vi "StreamProcess.Main.vi"(8 "error in (no error)":errorcluster, 9 "Refs":T1, 10 "FilterDVR.Ref":refnum<data-value>, 11 "Settings":T3) -> (0 "error out":errorcluster)   [LabVIEW 2025, in "xnet_can_bus_monitor_api_server_do.lvlib"]
uses:
  xnet_can_bus_monitor_api_server_do.lvlib
  Types/XNET.InitialSettings.ctl
  xnet_can_bus_monitor_api_server/RPC Messages/ni_xnet_can_bm_api_ConnectSettings.ctl
  xnet_can_bus_monitor_api_server/RPC Messages/ni_xnet_can_bm_api_CanMode.ctl
  xnet_can_bus_monitor_api_server/RPC Messages/ni_xnet_can_bm_api_Termination.ctl
  xnet_can_bus_monitor_api_server/RPC Messages/ni_xnet_can_bm_api_FdIsoMode.ctl
  xnet_can_bus_monitor_api_server/RPC Messages/ni_xnet_can_bm_api_FilterInfo.ctl
  xnet_can_bus_monitor_api_server/RPC Messages/ni_xnet_can_bm_api_DirectionFilter.ctl
  xnet_can_bus_monitor_api_server/RPC Messages/ni_xnet_can_bm_api_FrameFilter.ctl
  Types/StreamProcess.InputRefs.ctl
  <vilib>/gRPC/LabVIEW gRPC Library/Shared/grpcId.ctl
  Types/StreamProcess.State.ctl
  xnet_can_bus_monitor_api_server/RPC Messages/ni_xnet_can_bm_api_StreamBusReply.ctl
  xnet_can_bus_monitor_api_server/RPC Messages/ni_xnet_can_bm_api_CanCommState.ctl
  xnet_can_bus_monitor_api_server/RPC Messages/ni_xnet_can_bm_api_CommState.ctl
  xnet_can_bus_monitor_api_server/RPC Messages/ni_xnet_can_bm_api_LastCommError.ctl
  xnet_can_bus_monitor_api_server/RPC Messages/ni_xnet_can_bm_api_Frame.ctl
  xnet_can_bus_monitor_api_server/RPC Messages/ni_xnet_can_bm_api_ErrorInfo.ctl
  <vilib>/xnet/xnet.llb/XNET Create Session (Frame Input Stream).vi
  <vilib>/Utility/SystemLogging/Write to System Log.vi
  <vilib>/xnet/xnet.llb/XNET Read (Frame CAN).vi
  <vilib>/xnet/xnet.llb/XNET Read (State CAN Comm).vi
  <resource>/objmgr/xnet.rc
  xnet_can_bus_monitor_api_server/xnet_can_bus_monitor_api_server.lvlib
  xnet_can_bus_monitor_api_server/RPC Service/NI_XNET_CAN_Bus_Monitor_API/NI_XNET_CAN_Bus_Monitor_API.lvclass
  <vilib>/gRPC/LabVIEW gRPC Library/grpc-lvsupport-release.lvlib
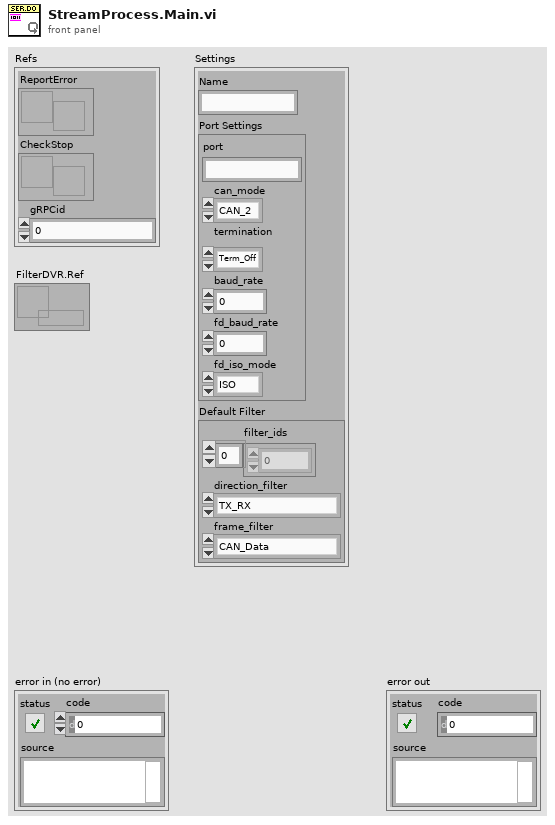
[diagram p1: front panel]
types:
  T1 = typedef "xnet_can_bus_monitor_api_server_do.lvlib/StreamProcess.InputRefs.ctl" = cluster{"ReportError":refnum<notifier>, "CheckStop":refnum<notifier>, "gRPCid":T2}
  T2 = typedef "grpc-lvsupport-release.lvlib/grpcId.ctl" = u64
  T3 = typedef "xnet_can_bus_monitor_api_server_do.lvlib/XNET.InitialSettings.ctl" = cluster{"Name":string, "Port Settings":T4, "Default Filter":T8}
  T4 = typedef "xnet_can_bus_monitor_api_server.lvlib/ni_xnet_can_bm_api_ConnectSettings.ctl" = cluster{"port":string, "can_mode":T5, "termination":T6, "baud_rate":u64, "fd_baud_rate":u64, "fd_iso_mode":T7}
  T5 = typedef "xnet_can_bus_monitor_api_server.lvlib/ni_xnet_can_bm_api_CanMode.ctl" = enum32{"CAN_2", "CAN_FD", "CAN_FD_BRS"}
  T6 = typedef "xnet_can_bus_monitor_api_server.lvlib/ni_xnet_can_bm_api_Termination.ctl" = enum32{"Term_Off", "Term_On"}
  T7 = typedef "xnet_can_bus_monitor_api_server.lvlib/ni_xnet_can_bm_api_FdIsoMode.ctl" = enum32{"ISO", "Non_ISO", "ISO_Legacy"}
  T8 = typedef "xnet_can_bus_monitor_api_server.lvlib/ni_xnet_can_bm_api_FilterInfo.ctl" = cluster{"filter_ids":u32[], "direction_filter":T9, "frame_filter":T10}
  T9 = typedef "xnet_can_bus_monitor_api_server.lvlib/ni_xnet_can_bm_api_DirectionFilter.ctl" = enum32{"TX_RX", "RX", "TX"}
  T10 = typedef "xnet_can_bus_monitor_api_server.lvlib/ni_xnet_can_bm_api_FrameFilter.ctl" = enum32{"CAN_Data", "CAN_Remote", "CAN_Bus_Error", "CAN_2_Data", "CAN_FD_Data", "CAN_FD_BRS_Data", "J1939_Data", "Delay", "Log_Trigger", "Start_Trigger", "All"}
  T11 = typedef "xnet_can_bus_monitor_api_server_do.lvlib/StreamProcess.State.ctl" = enum8{"Open XNET Session", "Publish", "Cleanup"}
  T12 = typedef "xnet_can_bus_monitor_api_server.lvlib/ni_xnet_can_bm_api_StreamBusReply.ctl" = cluster{"can_comm_state":T13, "frame":T16[], "error":T17}
  T13 = typedef "xnet_can_bus_monitor_api_server.lvlib/ni_xnet_can_bm_api_CanCommState.ctl" = cluster{"fault_code":i32, "fault":bool, "comm_state":T14, "last_comm_error":T15, "receive_error_counter":u32, "transmit_error_counter":u32, "transceiver_error":bool, "sleep":bool}
  T14 = typedef "xnet_can_bus_monitor_api_server.lvlib/ni_xnet_can_bm_api_CommState.ctl" = enum32{"Error_Active", "Error_Passive", "Bus_Off", "Init"}
  T15 = typedef "xnet_can_bus_monitor_api_server.lvlib/ni_xnet_can_bm_api_LastCommError.ctl" = enum32{"None", "Stuff", "Form", "ACK", "Bit1", "Bit0", "CRC"}
  T16 = typedef "xnet_can_bus_monitor_api_server.lvlib/ni_xnet_can_bm_api_Frame.ctl" = cluster{"timestamp":dbl, "payload":u8[], "identifier":u32, "frame_type":u32, "extended":bool, "echo":bool}
  T17 = typedef "xnet_can_bus_monitor_api_server.lvlib/ni_xnet_can_bm_api_ErrorInfo.ctl" = errorcluster
  T18 = typedef "XNET Frame CAN.ctl" = cluster{"timestamp":timestamp, "payload":u8[], "identifier":u32, "type":T19, "extended?":bool, "echo?":bool}
  T19 = typedef "XNET Frame Type CAN.ctl" = u8
  T20 = typedef "XNET CAN Comm.ctl" = cluster{"fault code":i32, "fault?":bool, "communication state":T21, "last error":T22, "receive error counter":u8, "transmit error counter":u8, "transceiver error?":bool, "sleep?":bool}
  T21 = typedef "XNET CAN Comm State.ctl" = u8
  T22 = typedef "XNET CAN Last Err.ctl" = u8
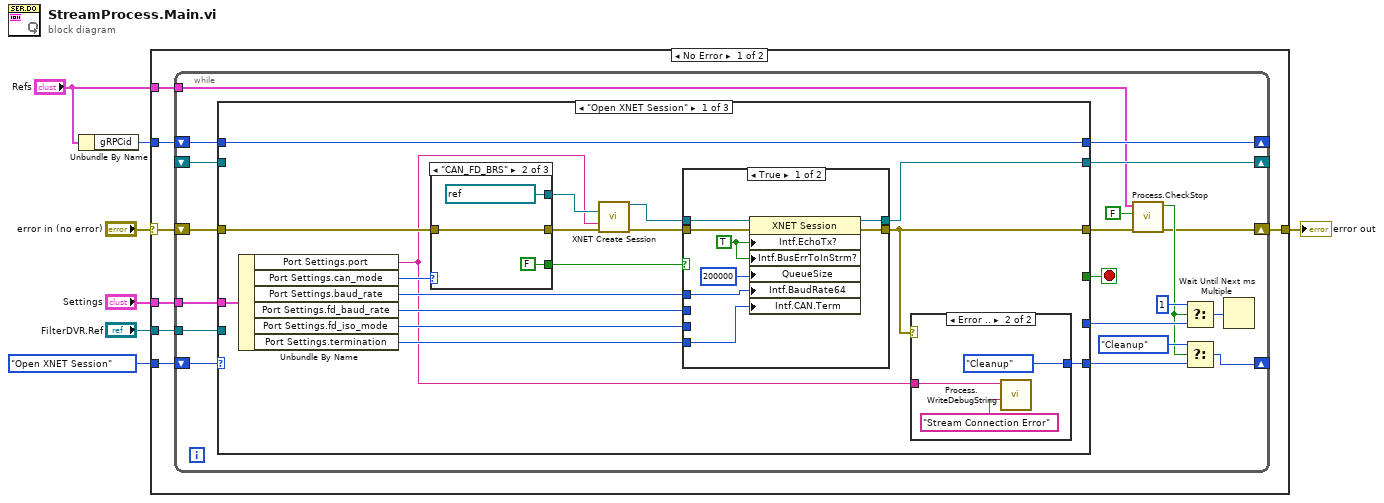
[diagram p0: block diagram]
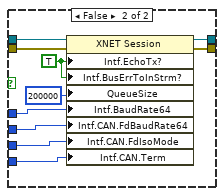
[diagram p2: hidden frame]
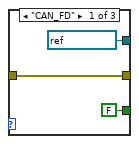
[diagram p3: hidden frame]
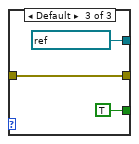
[diagram p4: hidden frame]
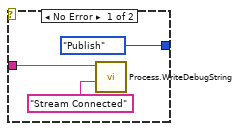
[diagram p5: hidden frame]
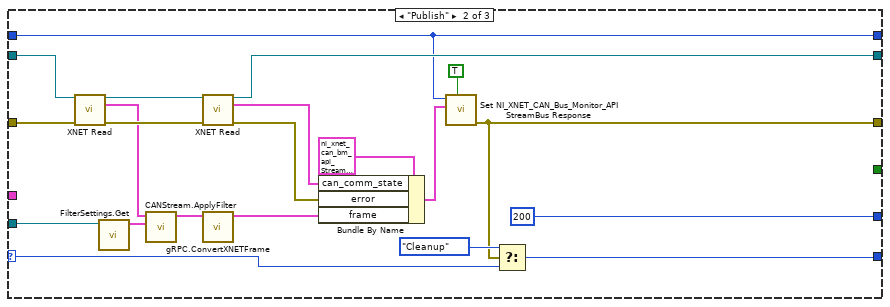
[diagram p6: hidden frame]
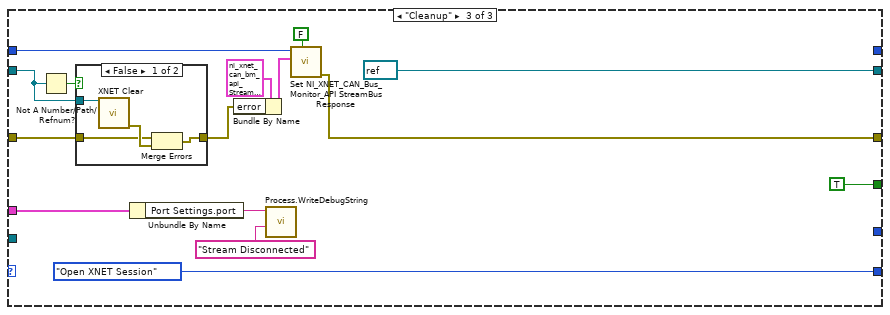
[diagram p7: hidden frame]
diagram:
  n1 = Unbundle By Name("Refs") -> ("gRPCid"=w1:T2)
  n2 = case shown="No Error" "error in (no error)" {
    selector: "error in (no error)" -> [w9 w126]
    tunnel: [w14 w126] -> w7
    tunnel: StreamProcess.State."Open XNET Session" -> [w13 _]
    tunnel: "Settings" -> [w12 _]
    tunnel: "Refs" -> [w11 _]
    tunnel: w1 -> [w10 _]
    tunnel: "FilterDVR.Ref" -> [w8 _]
    frame No Error {
      n3 = while {
        shift-right: [w24] -> _
        shift-left: w13 -> [w34]
        shift-right: [w33] -> _
        shift-left: w10 -> [w32]
        shift-right: [w16] -> w14
        shift-left: w9 -> [w31]
        shift-right: [w29] -> _
        shift-left: _ -> [w28]
        tunnel: w12 -> [w25]
        tunnel: w11 -> [w18]
        tunnel: w8 -> [w15]
        stop <- w30 stop-if-true
        n4 = case shown="\"Open XNET Session\"" w34 {
          selector: w34 -> [_ w105 _]
          tunnel: [w35 w104 StreamProcess.State."Open XNET Session"] -> w26
          tunnel: [w51 w91 _] -> w33
          tunnel: w32 -> [w51 w91 w111]
          tunnel: [w47 w90 w107] -> w17
          tunnel: w31 -> [w39 w100 w116]
          tunnel: [_ _ TRUE] -> w30
          tunnel: [w49 w97 refnum<k21> refnum ("session out")] -> w29
          tunnel: w28 -> [_ w102 w118]
          tunnel: [_ u32 200 ("millisecond multiple") _] -> w23
          tunnel: w25 -> [w46 _ w115]
          tunnel: w15 -> [_ w85 _]
          frame "Open XNET Session" {
            n5 = Unbundle By Name(w46) -> ("Port Settings.port"=w36:string, "Port Settings.can_mode"=w40:T5, "Port Settings.baud_rate"=w38:u64, "Port Settings.fd_baud_rate"=w37:u64, "Port Settings.fd_iso_mode"=w41:T7, "Port Settings.termination"=w45:T6)
            n6 = case shown="\"CAN_FD_BRS\"" w40 {
              tunnel: [refnum<k21> ":can_fd:" ("cluster (:memory:)") refnum<k21> ":can_fd_brs:" ("cluster (:memory:)") refnum<k21> ":memory:" ("cluster (:memory:)")] -> w44
              tunnel: w39 -> [w70 w73 w76]
              tunnel: [w70 w73 w76] -> w43
              tunnel: [FALSE FALSE TRUE] -> w42
              frame "CAN_FD" {
              }
              frame "CAN_FD_BRS" {
              }
              frame Default {
              }
            }
            n7 = call-poly <vilib>:"XNET Create Session.vi"("cluster (:memory:)"=w44, "interface"=w36, "error in (no error)"=w43) -> ("session out"=w50:refnum<k21>, "error out"=w48:errorcluster)  [unwired: 11 out]
            n8 = case shown="True" w42 {
              tunnel: w50 -> [w59 w69]
              tunnel: [w58 w68] -> w49
              tunnel: w48 -> [w57 w67]
              tunnel: [w56 w66] -> w47
              tunnel: w45 -> [w53 w63]
              tunnel: w38 -> [w52 w62]
              tunnel: w41 -> [_ w61]
              tunnel: w37 -> [_ w60]
              frame True {
                w54 = TRUE ("Interface:Echo Transmit?")
                n9 = property class="XNET Session"(reference=w59, error in=w57, "Intf.EchoTx?"=w54, "Intf.BusErrToInStrm?"=w54, "QueueSize"=u32 200000 ("Queue Size"), "Intf.BaudRate64"=w52, "Intf.CAN.Term"=w53) -> (reference out=w58:refnum<k21>, error out=w56:errorcluster)
              }
              frame False {
                w64 = TRUE ("Interface:Echo Transmit?")
                n10 = property class="XNET Session"(reference=w69, error in=w67, "Intf.EchoTx?"=w64, "Intf.BusErrToInStrm?"=w64, "QueueSize"=u32 200000 ("Queue Size"), "Intf.BaudRate64"=w62, "Intf.CAN.FdBaudRate64"=w60, "Intf.CAN.FdIsoMode"=w61, "Intf.CAN.Term"=w63) -> (reference out=w68:refnum<k21>, error out=w66:errorcluster)
              }
            }
            n11 = case shown="Error .." w47 {
              tunnel: w36 -> [w80 w83]
              tunnel: [StreamProcess.State."Publish" StreamProcess.State."Cleanup"] -> w35
              frame No Error {
                n12 = call "Process.WriteDebugString.vi"("State"="Stream Connected", "Name"=w80) -> ()  [unwired: 9 in, 1 out]
              }
              frame Error {
                n13 = call "Process.WriteDebugString.vi"("State"="Stream Connection Error", "Name"=w83) -> ()  [unwired: 9 in, 1 out]
              }
            }
          }
          frame "Publish" {
            n14 = call-poly <vilib>:"XNET Read.vi"("session in"=w102, "error in (no error)"=w100) -> ("session out"=w98:refnum<k21>, "data"=w95:T18[], "error out"=w99:errorcluster)  [unwired: 11 out]
            n15 = call "FilterSettings.Get.vi"("FilterDVR.Ref"=w85) -> ("Filter"=w94:T8)  [unwired: 9 in, 1 out]
            n16 = call "CANStream.ApplyFilter.vi"("Filter"=w94, "frames in"=w95) -> ("frames out"=w93:T18[])  [unwired: 9 in]
            n17 = call-poly <vilib>:"XNET Read.vi"("session in"=w98, "error in (no error)"=w99) -> ("session out"=w97:refnum<k21>, "CAN comm"=w96:T20, "error out"=w86:errorcluster)  [unwired: 11 out]
            n18 = call "gRPC.ConvertXNETFrame.vi"("frames in"=w93) -> ("Array"=w92:T16[])  [unwired: 10 in]
            n19 = Bundle By Name(cluster=T12 {"can_comm_state"={"fault_code"=0, "fault"=FALSE, "comm_state"=enum."Error_Active", "last_comm_error"=enum."None", "receive_error_counter"=0, "transmit_error_counter"=0, "transceiver_error"=FALSE, "sleep"=FALSE}, "frame"=[], "error"={"status"=FALSE, "code"=0, "source"=""}} ("Message Data"), "can_comm_state"=w96, "error"=w86, "frame"=w92) -> (w89:T12)
            n20 = call "Set NI_XNET_CAN_Bus_Monitor_API StreamBus Response.vi"("Streaming? (F)"=TRUE, "Message Data"=w89, "gRPCid in"=w91) -> ("error out"=w90:errorcluster)  [unwired: 8 in]
            n21 = Select(t=StreamProcess.State."Cleanup", s=w90, f=w105) -> (s? t:f=w104:T11)
          }
          frame "Cleanup" {
            n22 = Not A Number/Path/Refnum?(number/path/refnum=w118) -> (NaN/Path/Refnum?=w117:bool)
            n23 = case shown="False" w117 {
              tunnel: w116 -> [w121 w125]
              tunnel: [w122 w125] -> w108
              tunnel: w118 -> [w124 _]
              frame False {
                n24 = call <vilib>:"XNET Clear.vi"("session in"=w124) -> ("error out"=w123:errorcluster)  [unwired: 14 in]
                n25 = Merge Errors(w121, w123) -> (w122:errorcluster)
              }
              frame True {
              }
            }
            n26 = Unbundle By Name(w115) -> ("Port Settings.port"=w114:string)
            n27 = Bundle By Name(cluster=T12 {"can_comm_state"={"fault_code"=0, "fault"=FALSE, "comm_state"=enum."Error_Active", "last_comm_error"=enum."None", "receive_error_counter"=0, "transmit_error_counter"=0, "transceiver_error"=FALSE, "sleep"=FALSE}, "frame"=[], "error"={"status"=FALSE, "code"=0, "source"=""}} ("Message Data"), "error"=w108) -> (w109:T12)
            n28 = call "Process.WriteDebugString.vi"("State"="Stream Disconnected", "Name"=w114) -> ()  [unwired: 9 in, 1 out]
            n29 = call "Set NI_XNET_CAN_Bus_Monitor_API StreamBus Response.vi"("Streaming? (F)"=FALSE, "Message Data"=w109, "gRPCid in"=w111) -> ("error out"=w107:errorcluster)  [unwired: 8 in]
          }
        }
        n30 = call "Process.CheckStop.vi"("error in (no error)"=w17, "Stop Async on Error?"=FALSE, "LocalInterface.Refs"=w18) -> ("error out"=w16:errorcluster, "Stop"=w20:bool)  [unwired: 7 in]
        n31 = Select(t=u32 1, s=w20, f=w23) -> (s? t:f=w22:u32)
        n32 = Select(t=StreamProcess.State."Cleanup" ("y"), s=w20, f=w26) -> (s? t:f=w24:T11)
        n33 = Wait Until Next ms Multiple(millisecond multiple=w22) -> ()  [unwired: 1 out]
      }
    }
    frame Error {
    }
  }
  "error out" <- w7
